vi "MAX_DEVICES.vi"() -> (3 "MAX_DEVICES":i32=64)   [LabVIEW 2020, in "G-Audio.lvlib"]
uses:
  G-Audio.lvlib
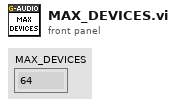
[diagram p1: front panel]
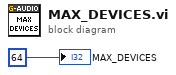
[diagram p0: block diagram]
diagram:
  "MAX_DEVICES" <- 64
